vi "MicroZed Read.vi"(8 "Error In":errorcluster, 11 "TCP Master Ref In":refnum<class "Modbus Master.lvclass">) -> (0 "Error Out":errorcluster, 2 "PC Data":T1 {"Alarms 2" format="%016b"; "Faults 2" format="%016b"; "Alarms 1" format="%016b"; "Faults 1" format="%016b"; "Contactor FB" format="%.0b"; "DC Voltage SP" format="%2.1f"; "Clear Faults SP" format="%.0b"; "Neutral Current" format="%2.1f"; "AC Current - L2" format="%2.1f"; "AC Voltage - L2" format="%2.1f"; "Temperature" format="%2.1f"; "DC Voltage" format="%2.1f"; "AC Current SP" format="%2.1f"; "AC Voltage SP" format="%2.1f"; "Frequency SP" format="%2.1f"; "AC Frequency" format="%2.1f"; "AC Current - L1" format="%2.1f"; "AC Voltage- L1" format="%2.1f"}, 3 "TCP Master Ref Out":refnum<class "Modbus Master.lvclass">)   [LabVIEW 2014]
uses:
  <vilib>/Modbus/master/Modbus Master.lvclass
  Controls/PC Data.ctl
  Controls/MicroZed Config Op Mode.ctl
  <vilib>/ptbypt/NI_PtbyPt.lvlib
panel:
  out "Negative Vdc":dbl format="%2.1f"
  out "Positive Vdc":dbl format="%2.1f"
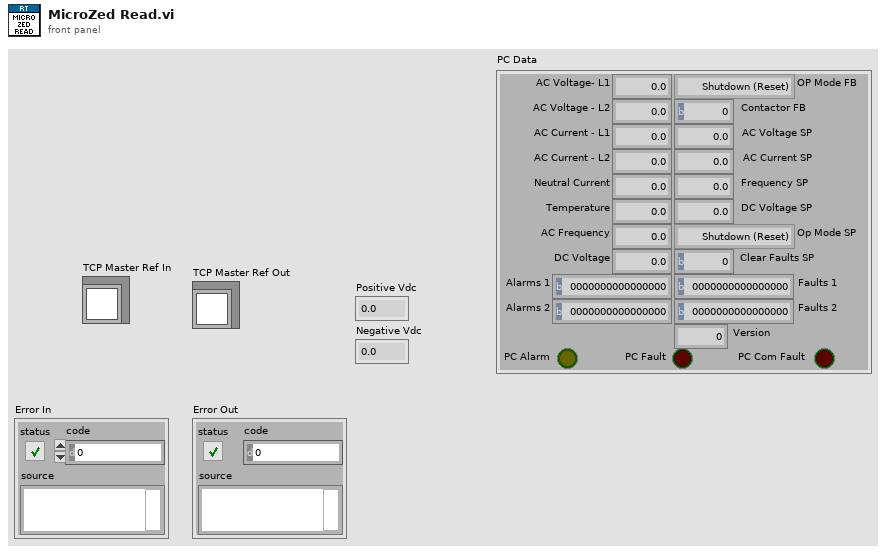
[diagram p1: front panel]
types:
  T1 = typedef "PC Data.ctl" = cluster{"AC Voltage- L1":dbl, "AC Voltage - L2":dbl, "AC Current - L1":dbl, "AC Current - L2":dbl, "Neutral Current":dbl, "Temperature":dbl, "AC Frequency":dbl, "DC Voltage":dbl, "AC Voltage SP":dbl, "AC Current SP":dbl, "Frequency SP":dbl, "Op Mode SP":T2, "Clear Faults SP":u16, "PC Com Fault":bool, "PC Fault":bool, "DC Voltage SP":dbl, "OP Mode FB":T2, "Contactor FB":u16, "Faults 1":u16, "Alarms 1":u16, "Faults 2":u16, "Alarms 2":u16, "PC Alarm":bool, "Version":u16}
  T2 = typedef "MicroZed Config Op Mode.ctl" = enum16{"Shutdown (Reset)", "Startup", "Idle", "Voltage Mode", "Current Mode", "Fault", "OL Voltage (Debug)", "No Data"}
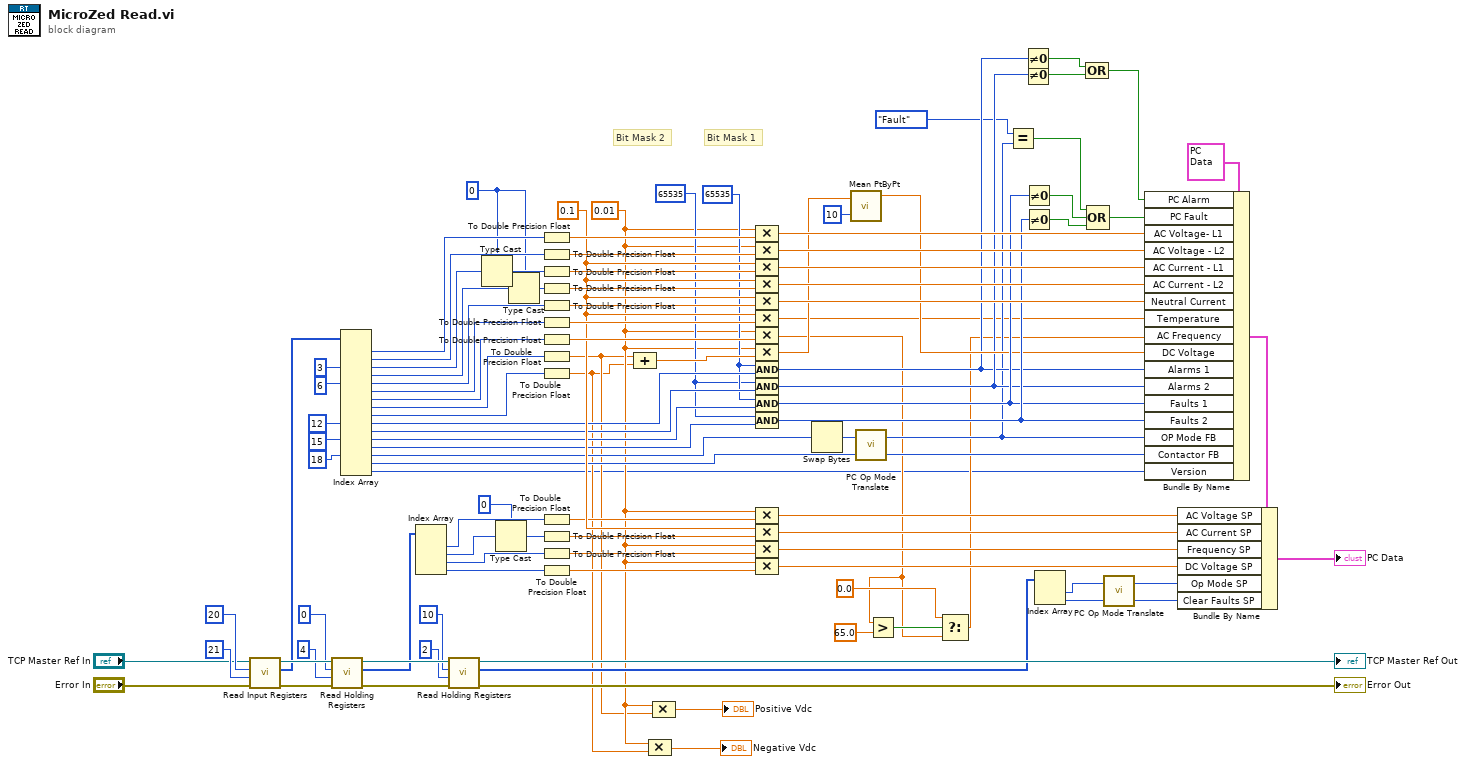
[diagram p0: block diagram]
diagram:
  w21 = i16 0
  w40 = u16 65535 ("value")
  w39 = u16 65535 ("value")
  w58 = 0.1 ("y")
  w13 = 0.01 ("y")
  # "Bit Mask 1"
  # "Bit Mask 2"
  n1 = call-dynamic "Read Input Registers.vi"("error in (no error)"="Error In", "number of input registers"=u16 21 ("number of holding registers"), "starting address"=u16 20, "Modbus master in"="TCP Master Ref In") -> ("error out"=w100:errorcluster, "register values"=w75:u16[], "Modbus master out"=w97:refnum<class "Modbus Master.lvclass">)  [unwired: 5 in]
  n2 = call-dynamic "Read Holding Registers.vi"("error in (no error)"=w100, "number of holding registers"=u16 4, "starting address"=u16 0, "Modbus master in"=w97) -> ("error out"=w99:errorcluster, "register values"=w30:u16[], "Modbus master out"=w96:refnum<class "Modbus Master.lvclass">)  [unwired: 5 in]
  n3 = Index Array(array=w75, index #3=3 ("index"), index #5=6 ("index"), index #10=12 ("index"), index #12=15 ("index"), index #14=18 ("index")) -> (element #1=w90:u16, element #2=w88:u16, element #3=w86:u16, element #4=w85:u16, element #5=w84:u16, element #6=w80:u16, element #7=w67:u16, element #8=w54:u16, element #9=w48:u16, element #10=w45:u16, element #11=w44:u16, element #12=w43:u16, element #13=w42:u16, element #14=w41:u16, element #15=w36:u16, element #16=w1:u16)  [unwired: 11 in]
  n4 = Index Array(array=w30) -> (element #1=w62:u16, element #2=w59:u16, element #3=w60:u16, element #4=w61:u16)  [unwired: 4 in]
  n5 = call-dynamic "Read Holding Registers.vi"("error in (no error)"=w99, "number of holding registers"=u16 2, "starting address"=u16 10, "Modbus master in"=w96) -> ("error out"=→"Error Out":errorcluster, "register values"=w81:u16[], "Modbus master out"=→"TCP Master Ref Out":refnum<class "Modbus Master.lvclass">)  [unwired: 5 in]
  n6 = Type Cast(type=w21, x=w86) -> (*(type *) &x=w23:i16)
  n7 = Type Cast(type=i16 0, x=w59) -> (*(type *) &x=w25:i16)
  n8 = Type Cast(type=w21, x=w85) -> (*(type *) &x=w22:i16)
  n9 = To Double Precision Float(number=w90) -> (double precision float=w69:dbl)
  n10 = To Double Precision Float(number=w88) -> (double precision float=w70:dbl)
  n11 = To Double Precision Float(number=w23) -> (double precision float=w71:dbl)
  n12 = To Double Precision Float(number=w22) -> (double precision float=w72:dbl)
  n13 = To Double Precision Float(number=w84) -> (double precision float=w73:dbl)
  n14 = To Double Precision Float(number=w80) -> (double precision float=w74:dbl)
  n15 = To Double Precision Float(number=w67) -> (double precision float=w66:dbl)
  n16 = To Double Precision Float(number=w54) -> (double precision float=w12:dbl)
  n17 = To Double Precision Float(number=w48) -> (double precision float=w11:dbl)
  n18 = To Double Precision Float(number=w62) -> (double precision float=w29:dbl)
  n19 = To Double Precision Float(number=w25) -> (double precision float=w26:dbl)
  n20 = To Double Precision Float(number=w60) -> (double precision float=w28:dbl)
  n21 = To Double Precision Float(number=w61) -> (double precision float=w27:dbl)
  n22 = Compound Arithmetic op=ADD(w12, w11) -> (w47:dbl)
  n23 = Compound Arithmetic op=MULTIPLY(w13, w11) -> (→"Negative Vdc":dbl)
  n24 = Compound Arithmetic op=MULTIPLY(w13, w12) -> (→"Positive Vdc":dbl)
  n25 = Compound Arithmetic op=MULTIPLY(w13, w69) -> (w89:dbl)
  n26 = Compound Arithmetic op=MULTIPLY(w13, w70) -> (w87:dbl)
  n27 = Compound Arithmetic op=MULTIPLY(w58, w71) -> (w79:dbl)
  n28 = Compound Arithmetic op=MULTIPLY(w58, w72) -> (w77:dbl)
  n29 = Compound Arithmetic op=MULTIPLY(w58, w73) -> (w76:dbl)
  n30 = Compound Arithmetic op=MULTIPLY(w58, w74) -> (w3:dbl)
  n31 = Compound Arithmetic op=MULTIPLY(w13, w66) -> (w4:dbl)
  n32 = Compound Arithmetic op=MULTIPLY(w13, w47) -> (w32:dbl)
  n33 = Compound Arithmetic op=AND(w40, w45) -> (w16:u16)
  n34 = Compound Arithmetic op=AND(w39, w44) -> (w17:u16)
  n35 = Compound Arithmetic op=AND(w40, w43) -> (w49:u16)
  n36 = Compound Arithmetic op=AND(w39, w42) -> (w50:u16)
  n37 = Compound Arithmetic op=MULTIPLY(w13, w29) -> (w65:dbl)
  n38 = Compound Arithmetic op=MULTIPLY(w58, w26) -> (w64:dbl)
  n39 = Compound Arithmetic op=MULTIPLY(w13, w28) -> (w63:dbl)
  n40 = Compound Arithmetic op=MULTIPLY(w13, w27) -> (w34:dbl)
  n41 = Swap Bytes(anything=w41) -> (byte swapped=w35:u16)
  n42 = call <vilib>:"Mean PtByPt.vi"("x"=w32, "sample length"=10) -> ("mean"=w31:dbl)  [unwired: 2 in, 1 out]
  n43 = call "PC Op Mode Translate.vi"("Op Mode In"=w35) -> ("Op Mode Out"=w14:T2)  [unwired: 2 in]
  n44 = Greater?(x=w4, y=65.0) -> (0:w7:bool)
  n45 = Select(t=0.0, s=w7, f=w4) -> (s? t:f=w5:dbl)
  n46 = Equal?(x=MicroZed_Config_Op_Mode."Fault" ("Op Mode Out"), y=w14) -> (x = y?=w2:bool)
  n47 = Not Equal To 0?(x=w16) -> (x != 0?=w19:bool)
  n48 = Not Equal To 0?(x=w17) -> (x != 0?=w20:bool)
  n49 = Not Equal To 0?(x=w49) -> (x != 0?=w52:bool)
  n50 = Not Equal To 0?(x=w50) -> (x != 0?=w53:bool)
  n51 = Index Array(array=w81) -> (element #1=w56:u16, element #2=w57:u16)  [unwired: 2 in]
  n52 = Compound Arithmetic op=OR(w19, w20) -> (w18:bool)
  n53 = Compound Arithmetic op=OR(w2, w52, w53) -> (w51:bool)
  n54 = call "PC Op Mode Translate.vi"("Op Mode In"=w56) -> ("Op Mode Out"=w55:T2)  [unwired: 2 in]
  n55 = Bundle By Name(cluster=T1 {"AC Voltage- L1"=0.0, "AC Voltage - L2"=0.0, "AC Current - L1"=0.0, "AC Current - L2"=0.0, "Neutral Current"=0.0, "Temperature"=0.0, "AC Frequency"=0.0, "DC Voltage"=0.0, "AC Voltage SP"=0.0, "AC Current SP"=0.0, "Frequency SP"=0.0, "Op Mode SP"=enum."Shutdown (Reset)", "Clear Faults SP"=0, "PC Com Fault"=FALSE, "PC Fault"=FALSE, "DC Voltage SP"=0.0, "OP Mode FB"=enum."Shutdown (Reset)", "Contactor FB"=0, "Faults 1"=0, "Alarms 1"=0, "Faults 2"=0, "Alarms 2"=0, "PC Alarm"=FALSE, "Version"=0} ("PC Data"), "PC Alarm"=w18, "PC Fault"=w51, "AC Voltage- L1"=w89, "AC Voltage - L2"=w87, "AC Current - L1"=w79, "AC Current - L2"=w77, "Neutral Current"=w76, "Temperature"=w3, "AC Frequency"=w5, "DC Voltage"=w31, "Alarms 1"=w16, "Alarms 2"=w17, "Faults 1"=w49, "Faults 2"=w50, "OP Mode FB"=w14, "Contactor FB"=w36, "Version"=w1) -> (w83:T1)
  n56 = Bundle By Name(cluster=w83, "AC Voltage SP"=w65, "AC Current SP"=w64, "Frequency SP"=w63, "DC Voltage SP"=w34, "Op Mode SP"=w55, "Clear Faults SP"=w57) -> (→"PC Data":T1)
